vi "z.stack.configure_MD.vi"() -> ()   [LabVIEW 2012]
uses:
  GFG/GFGnumericGet.vi
  GFG/GFGbooleanGet.vi
  GFG/GFG library.lvlib
  GFG/GFGfpRefGet.vi
panel:
  in  "error in (no error)":errorcluster
  out "error out":errorcluster
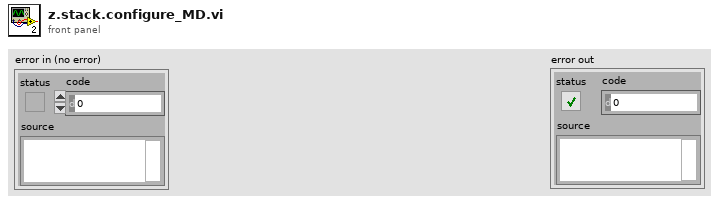
[diagram p1: front panel]
types:
  T1 = cluster{"WaveformChartRef":refnum<vi>, "DigitalRef":refnum<vi>, "ArrayRef":refnum<vi>, "TabControlRef":refnum<vi>, "EnumRef":refnum<vi>, "RingRef":refnum<vi>, "BooleanRef":refnum<vi>, "KnobRef":refnum<vi>, "SlideRef":refnum<vi>, "PathRef":refnum<vi>, "StringRef":refnum<vi>, "ComboBox":refnum<vi>, "WaveformGraphRef":refnum<vi>}
  T2 = enum8{"Enabled", "Disabled", "Disabled and Grayed Out"}
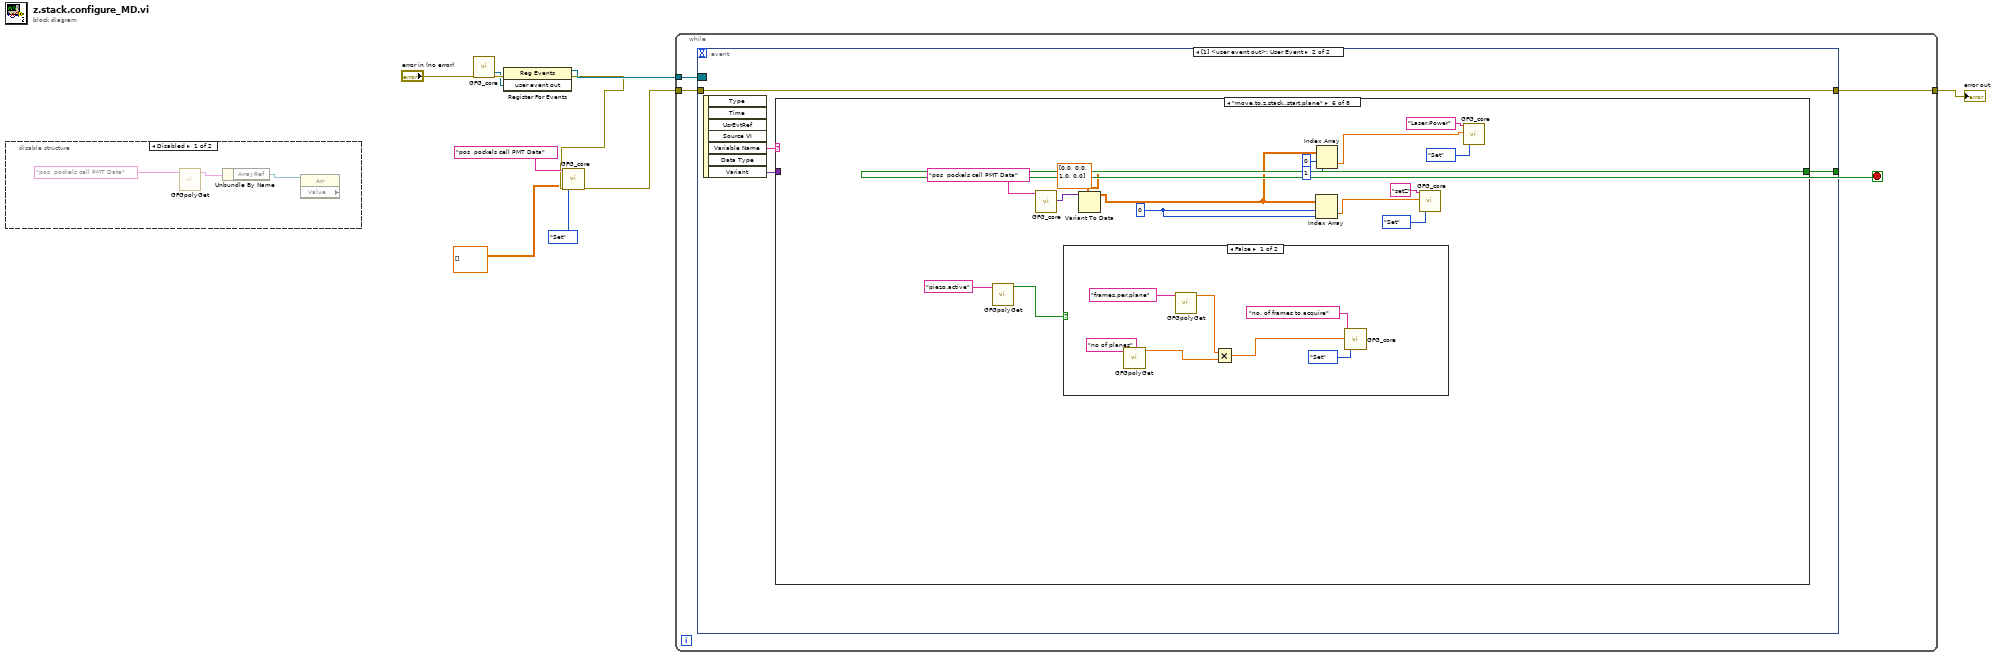
[diagram p0: block diagram]
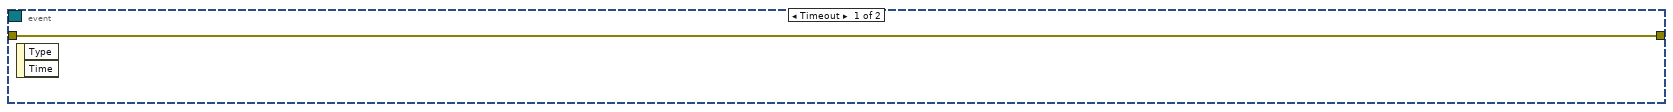
[diagram p3: hidden frame]
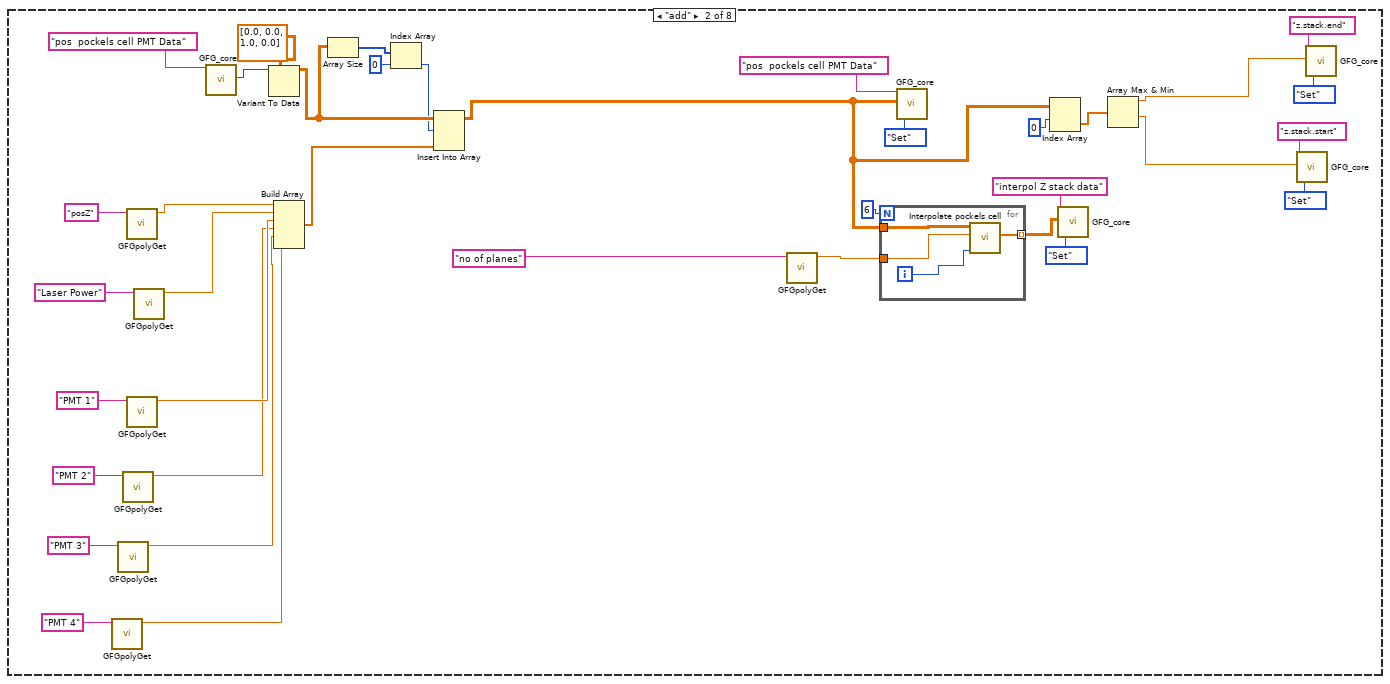
[diagram p5: hidden frame]
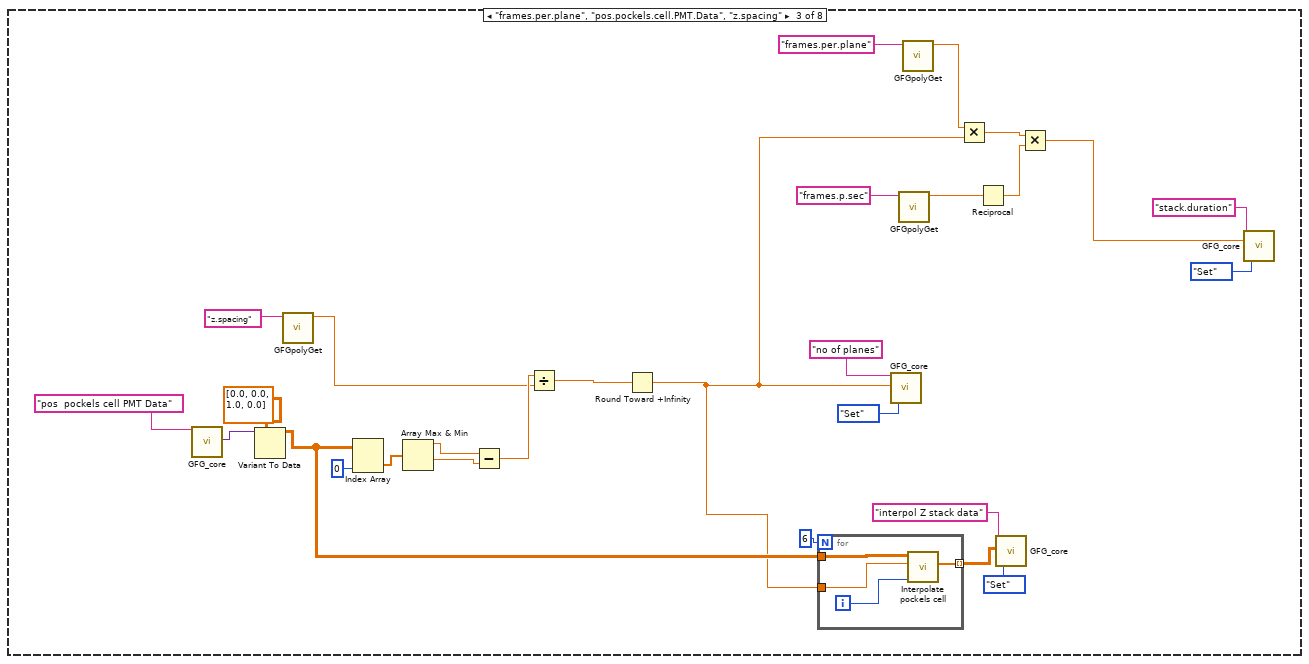
[diagram p6: hidden frame]
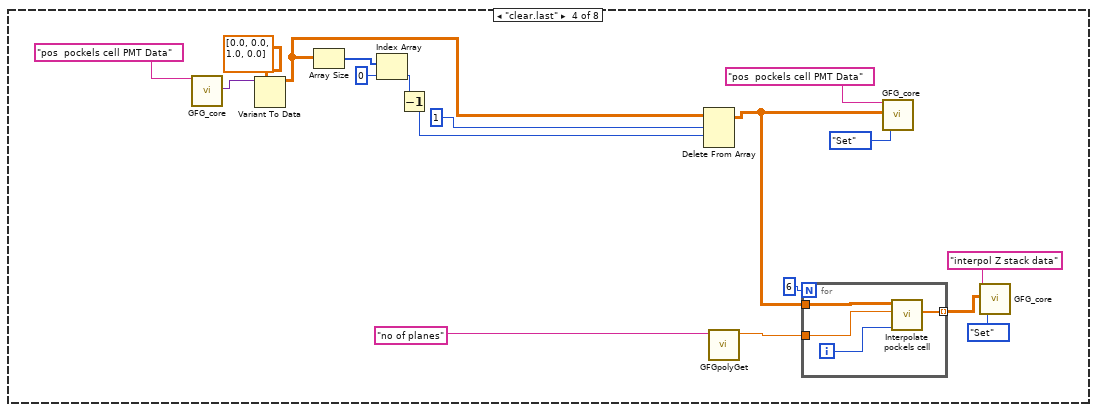
[diagram p7: hidden frame]
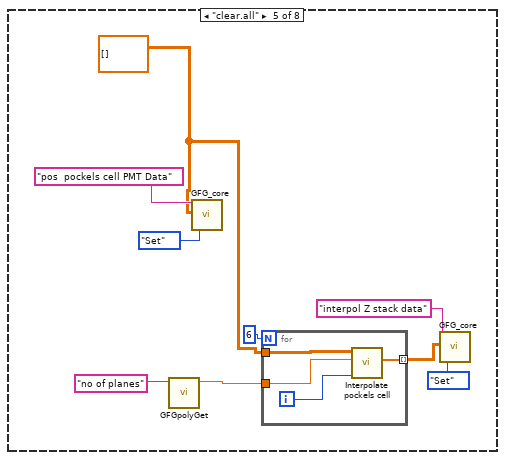
[diagram p8: hidden frame]
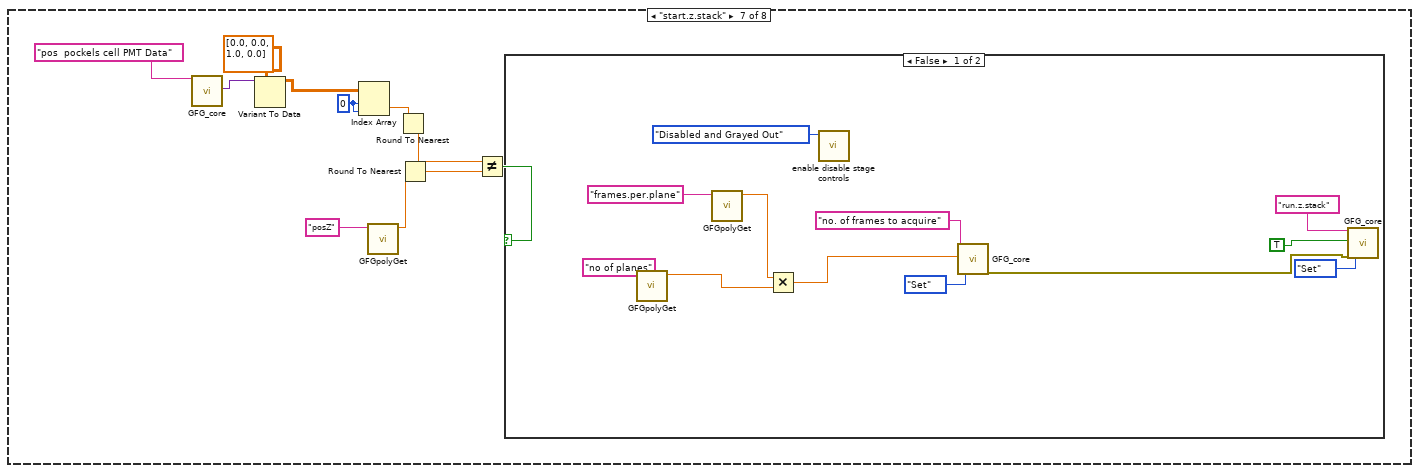
[diagram p10: hidden frame]
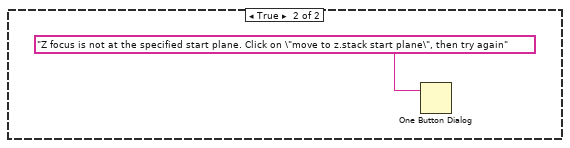
[diagram p11: hidden frame]
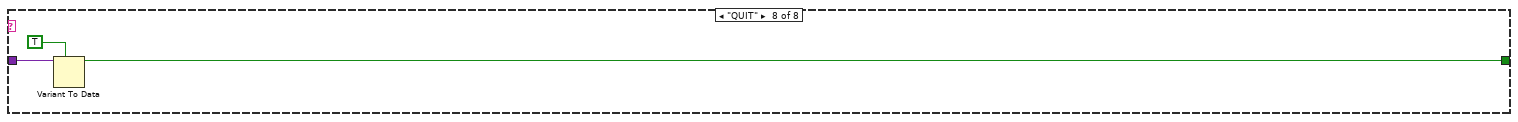
[diagram p12: hidden frame]
diagram:
  n1 = disable-structure shown="Disabled" {
    frame Disabled {
      n2 = call-poly "GFGpolyGet.vi"("Variable Name in"="pos  pockels cell PMT Data") -> ("output cluster"=w12:T1)  [unwired: 9 in, 1 out]
      n3 = Unbundle By Name(w12) -> ("ArrayRef"=w11:refnum<vi>)
      n4 = property class="Arr" props=["Value"](reference=w11) -> ()  [unwired: 1 in, 3 out]
    }
    frame Enabled {
    }
  }
  n5 = call "GFG_core.vi"("error in (no error)"="error in (no error)") -> ("user event out"=w7:refnum<user-event>, "error out"=w8:errorcluster)  [unwired: 12 in, 5 out]
  n6 = register-events(error in=w8, w7) -> (reference out=w6:refnum<event-registration>, error out=w4:errorcluster)  [unwired: 1 in]
  n7 = call "GFG_core.vi"("Variable Name in"="pos  pockels cell PMT Data", "Variant in"=dbl[][] [] ("output array"), "error in (no error)"=w4, "Action"=enum16{"Init", "Set", "Get"}."Set") -> ("error out"=w2:errorcluster)  [unwired: 9 in, 6 out]
  n8 = while {
    tunnel: w6 -> [w17]
    tunnel: w2 -> [w15]
    tunnel: [w14] -> w10
    stop <- w16 stop-if-true
    n9 = event shown="[1] <user event out>: User Event" {
      selector: w17 -> [_ _]
      dyn-events: _ -> [_ _]
      timeout: _ -> [_ _]
      tunnel: [_ w20] -> w16
      tunnel: w15 -> [w18 w19]
      tunnel: [w18 w19] -> w14
      event Timeout {
        n10 = event-data() -> ()  [unwired: 1 in, 2 out]
      }
      event User Event {
        n11 = event-data() -> ("Variable Name"=w22:string, "Variant"=w21:variant)  [unwired: 1 in, 5 out]
        n12 = case shown="\"move.to.z.stack..start.plane\"" w22 {
          tunnel: w21 -> [_ _ _ _ _ _ _ w179]
          tunnel: [_ _ _ _ _ _ _ w177] -> w20
          frame "False", Default {
          }
          frame "add" {
            n13 = call-poly "GFGpolyGet.vi"("Variable Name in"="PMT 4") -> ("Numeric"=w41:dbl)  [unwired: 9 in, 1 out]
            n14 = call-poly "GFGpolyGet.vi"("Variable Name in"="PMT 3") -> ("Numeric"=w42:dbl)  [unwired: 9 in, 1 out]
            n15 = call-poly "GFGpolyGet.vi"("Variable Name in"="PMT 2") -> ("Numeric"=w43:dbl)  [unwired: 9 in, 1 out]
            n16 = call-poly "GFGpolyGet.vi"("Variable Name in"="posZ") -> ("Numeric"=w46:dbl)  [unwired: 9 in, 1 out]
            n17 = call-poly "GFGpolyGet.vi"("Variable Name in"="PMT 1") -> ("Numeric"=w44:dbl)  [unwired: 9 in, 1 out]
            n18 = call-poly "GFGpolyGet.vi"("Variable Name in"="Laser Power") -> ("Numeric"=w45:dbl)  [unwired: 9 in, 1 out]
            n19 = call "GFG_core.vi"("Variable Name in"="pos  pockels cell PMT Data") -> ("Variant Out"=w58:variant)  [unwired: 12 in, 6 out]
            n20 = Variant To Data(type=dbl[][] [[0.0, 0.0], [1.0, 0.0]] ("pos  pockels cell PMT Data"), Variant=w58) -> (data=w56:dbl[][])  [unwired: 1 in, 1 out]
            n21 = Build Array(w46, w45, w44, w43, w42, w41) -> (w40:dbl[])
            n22 = Array Size(array=w56) -> (size(s)=w55:i32[])
            n23 = Index Array(array=w55, index=0) -> (element=w53:i32)
            n24 = Insert Into Array(array=w56, index (row)=w53, new element=w40) -> (w29:dbl[][])  [unwired: 1 in]
            n25 = call-poly "GFGpolyGet.vi"("Variable Name in"="no of planes") -> ("Numeric"=w35:dbl)  [unwired: 9 in, 1 out]
            n26 = for {
              N: 6 -> [_]
              tunnel: w29 -> [w63]
              tunnel: w35 -> [w62]
              tunnel: [w61] -> w32 mode=indexing
              i -> [w60]
              n27 = call "Interpolate pockels cell.vi"("column"=w60, "nr of planes"=w62, "Data"=w63) -> ("Interpolated Data"=w61:dbl[])  [unwired: 7 in, 1 out]
            }
            n28 = call "GFG_core.vi"("Variable Name in"="pos  pockels cell PMT Data", "Variant in"=w29, "Action"=enum16{"Init", "Set", "Get"}."Set") -> ()  [unwired: 10 in, 7 out]
            n29 = Index Array(array=w29, index (row)=0 ("disabled index (col)")) -> (element=w31:dbl[])  [unwired: 1 in]
            n30 = call "GFG_core.vi"("Variable Name in"="interpol Z stack data", "Variant in"=w32, "Action"=enum16{"Init", "Set", "Get"}."Set") -> ()  [unwired: 10 in, 7 out]
            n31 = Array Max & Min(array=w31) -> (max value=w23:dbl, min value=w24:dbl)  [unwired: 2 out]
            n32 = call "GFG_core.vi"("Variable Name in"="z.stack.start", "Variant in"=w24, "Action"=enum16{"Init", "Set", "Get"}."Set") -> ()  [unwired: 10 in, 7 out]
            n33 = call "GFG_core.vi"("Variable Name in"="z.stack.end", "Variant in"=w23, "Action"=enum16{"Init", "Set", "Get"}."Set") -> ()  [unwired: 10 in, 7 out]
          }
          frame "frames.per.plane", "pos.pockels.cell.PMT.Data", "z.spacing" {
            n34 = call "GFG_core.vi"("Variable Name in"="pos  pockels cell PMT Data") -> ("Variant Out"=w77:variant)  [unwired: 12 in, 6 out]
            n35 = Variant To Data(type=dbl[][] [[0.0, 0.0], [1.0, 0.0]] ("pos  pockels cell PMT Data"), Variant=w77) -> (data=w69:dbl[][])  [unwired: 1 in, 1 out]
            n36 = call-poly "GFGpolyGet.vi"("Variable Name in"="z.spacing") -> ("Numeric"=w67:dbl)  [unwired: 9 in, 1 out]
            n37 = Index Array(array=w69, index (col)=0 ("disabled index (col)")) -> (element=w79:dbl[])  [unwired: 1 in]
            n38 = Array Max & Min(array=w79) -> (max value=w81:dbl, min value=w82:dbl)  [unwired: 2 out]
            n39 = Subtract(x=w81, y=w82) -> (x-y=w75:dbl)
            n40 = Divide(x=w75, y=w67) -> (x/y=w74:dbl)
            n41 = Round Toward +Infinity(x=w74) -> (ceil(x): smallest int >= x=w64:dbl)
            n42 = for {
              N: 6 -> [_]
              tunnel: w69 -> [w95]
              tunnel: w64 -> [w94]
              tunnel: [w93] -> w70 mode=indexing
              i -> [w92]
              n43 = call "Interpolate pockels cell.vi"("column"=w92, "nr of planes"=w94, "Data"=w95) -> ("Interpolated Data"=w93:dbl[])  [unwired: 7 in, 1 out]
            }
            n44 = call "GFG_core.vi"("Variable Name in"="no of planes", "Variant in"=w64, "Action"=enum16{"Init", "Set", "Get"}."Set") -> ()  [unwired: 10 in, 7 out]
            n45 = call-poly "GFGpolyGet.vi"("Variable Name in"="frames.p.sec") -> ("Numeric"=w90:dbl)  [unwired: 9 in, 1 out]
            n46 = call-poly "GFGpolyGet.vi"("Variable Name in"="frames.per.plane") -> ("Numeric"=w65:dbl)  [unwired: 9 in, 1 out]
            n47 = Multiply(x=w65, y=w64) -> (x*y=w88:dbl)
            n48 = Reciprocal(x=w90) -> (1/x=w89:dbl)
            n49 = call "GFG_core.vi"("Variable Name in"="interpol Z stack data", "Variant in"=w70, "Action"=enum16{"Init", "Set", "Get"}."Set") -> ()  [unwired: 10 in, 7 out]
            n50 = Multiply(x=w88, y=w89) -> (x*y=w85:dbl)
            n51 = call "GFG_core.vi"("Variable Name in"="stack.duration", "Variant in"=w85, "Action"=enum16{"Init", "Set", "Get"}."Set") -> ()  [unwired: 10 in, 7 out]
          }
          frame "clear.last" {
            n52 = call "GFG_core.vi"("Variable Name in"="pos  pockels cell PMT Data") -> ("Variant Out"=w112:variant)  [unwired: 12 in, 6 out]
            n53 = Variant To Data(type=dbl[][] [[0.0, 0.0], [1.0, 0.0]] ("pos  pockels cell PMT Data"), Variant=w112) -> (data=w110:dbl[][])  [unwired: 1 in, 1 out]
            n54 = Array Size(array=w110) -> (size(s)=w109:i32[])
            n55 = Index Array(array=w109, index=0) -> (element=w105:i32)
            n56 = Decrement(x=w105) -> (x-1=w104:i32)
            n57 = Delete From Array(array=w110, length=1, index (row)=w104) -> (array with subset deleted=w96:dbl[][])  [unwired: 1 in, 1 out]
            n58 = call-poly "GFGpolyGet.vi"("Variable Name in"="no of planes") -> ("Numeric"=w100:dbl)  [unwired: 9 in, 1 out]
            n59 = for {
              N: 6 -> [_]
              tunnel: w96 -> [w117]
              tunnel: w100 -> [w116]
              tunnel: [w115] -> w97 mode=indexing
              i -> [w114]
              n60 = call "Interpolate pockels cell.vi"("column"=w114, "nr of planes"=w116, "Data"=w117) -> ("Interpolated Data"=w115:dbl[])  [unwired: 7 in, 1 out]
            }
            n61 = call "GFG_core.vi"("Variable Name in"="pos  pockels cell PMT Data", "Variant in"=w96, "Action"=enum16{"Init", "Set", "Get"}."Set") -> ()  [unwired: 10 in, 7 out]
            n62 = call "GFG_core.vi"("Variable Name in"="interpol Z stack data", "Variant in"=w97, "Action"=enum16{"Init", "Set", "Get"}."Set") -> ()  [unwired: 10 in, 7 out]
          }
          frame "clear.all" {
            w118 = dbl[][] [] ("output array")
            n63 = call-poly "GFGpolyGet.vi"("Variable Name in"="no of planes") -> ("Numeric"=w122:dbl)  [unwired: 9 in, 1 out]
            n64 = call "GFG_core.vi"("Variable Name in"="pos  pockels cell PMT Data", "Variant in"=w118, "Action"=enum16{"Init", "Set", "Get"}."Set") -> ()  [unwired: 10 in, 7 out]
            n65 = for {
              N: 6 -> [_]
              tunnel: w118 -> [w130]
              tunnel: w122 -> [w129]
              tunnel: [w128] -> w119 mode=indexing
              i -> [w127]
              n66 = call "Interpolate pockels cell.vi"("column"=w127, "nr of planes"=w129, "Data"=w130) -> ("Interpolated Data"=w128:dbl[])  [unwired: 7 in, 1 out]
            }
            n67 = call "GFG_core.vi"("Variable Name in"="interpol Z stack data", "Variant in"=w119, "Action"=enum16{"Init", "Set", "Get"}."Set") -> ()  [unwired: 10 in, 7 out]
          }
          frame "move.to.z.stack..start.plane" {
            w142 = 0 ("index (row)")
            n68 = call-poly "GFGpolyGet.vi"("Variable Name in"="piezo.active") -> ("Boolean"=w137:bool)  [unwired: 10 in]
            n69 = call "GFG_core.vi"("Variable Name in"="pos  pockels cell PMT Data") -> ("Variant Out"=w144:variant)  [unwired: 12 in, 6 out]
            n70 = case shown="False" w137 {
              frame False {
                n71 = call-poly "GFGpolyGet.vi"("Variable Name in"="no of planes") -> ("Numeric"=w151:dbl)  [unwired: 9 in, 1 out]
                n72 = call-poly "GFGpolyGet.vi"("Variable Name in"="frames.per.plane") -> ("Numeric"=w149:dbl)  [unwired: 9 in, 1 out]
                n73 = Multiply(x=w149, y=w151) -> (x*y=w152:dbl)
                n74 = call "GFG_core.vi"("Variable Name in"="no. of frames to acquire", "Variant in"=w152, "Action"=enum16{"Init", "Set", "Get"}."Set") -> ()  [unwired: 10 in, 7 out]
              }
              frame True {
              }
            }
            n75 = Variant To Data(type=dbl[][] [[0.0, 0.0], [1.0, 0.0]] ("pos  pockels cell PMT Data"), Variant=w144) -> (data=w134:dbl[][])  [unwired: 1 in, 1 out]
            n76 = Index Array(array=w134, index (row)=w142, index (col)=w142) -> (element=w139:dbl)
            n77 = Index Array(array=w134, index (row)=0, index (col)=1 ("disabled index (col)")) -> (element=w131:dbl)
            n78 = call "GFG_core.vi"("Variable Name in"="setZ", "Variant in"=w139, "Action"=enum16{"Init", "Set", "Get"}."Set") -> ()  [unwired: 10 in, 7 out]
            n79 = call "GFG_core.vi"("Variable Name in"="Laser.Power", "Variant in"=w131, "Action"=enum16{"Init", "Set", "Get"}."Set") -> ()  [unwired: 10 in, 7 out]
          }
          frame "start.z.stack" {
            w159 = 0 ("index (row)")
            n80 = call "GFG_core.vi"("Variable Name in"="pos  pockels cell PMT Data") -> ("Variant Out"=w162:variant)  [unwired: 12 in, 6 out]
            n81 = Variant To Data(type=dbl[][] [[0.0, 0.0], [1.0, 0.0]] ("pos  pockels cell PMT Data"), Variant=w162) -> (data=w160:dbl[][])  [unwired: 1 in, 1 out]
            n82 = Index Array(array=w160, index (row)=w159, index (col)=w159) -> (element=w157:dbl)
            n83 = call-poly "GFGpolyGet.vi"("Variable Name in"="posZ") -> ("Numeric"=w156:dbl)  [unwired: 9 in, 1 out]
            n84 = Round To Nearest(number=w157) -> (nearest integer value=w154:dbl)
            n85 = Round To Nearest(number=w156) -> (nearest integer value=w153:dbl)
            n86 = Not Equal?(x=w154, y=w153) -> (x != y?=w155:bool)
            n87 = case shown="False" w155 {
              frame False {
                n88 = call-poly "GFGpolyGet.vi"("Variable Name in"="no of planes") -> ("Numeric"=w170:dbl)  [unwired: 9 in, 1 out]
                n89 = call-poly "GFGpolyGet.vi"("Variable Name in"="frames.per.plane") -> ("Numeric"=w168:dbl)  [unwired: 9 in, 1 out]
                n90 = Multiply(x=w168, y=w170) -> (x*y=w171:dbl)
                n91 = call "enable disable stage controls.vi"("Disabled"=T2."Disabled and Grayed Out") -> ()  [unwired: 11 in]
                n92 = call "GFG_core.vi"("Variable Name in"="no. of frames to acquire", "Variant in"=w171, "Action"=enum16{"Init", "Set", "Get"}."Set") -> ("error out"=w164:errorcluster)  [unwired: 10 in, 6 out]
                n93 = call "GFG_core.vi"("Variable Name in"="run.z.stack", "Variant in"=TRUE, "error in (no error)"=w164, "Action"=enum16{"Init", "Set", "Get"}."Set") -> ()  [unwired: 9 in, 7 out]
              }
              frame True {
                n94 = One Button Dialog(message="Z focus is not at the specified start plane. Click on \"move to z.stack start plane\", then try again") -> ()  [unwired: 1 in, 1 out]
              }
            }
          }
          frame "QUIT" {
            n95 = Variant To Data(type=TRUE ("want seconds? (F)"), Variant=w179) -> (data=w177:bool)  [unwired: 1 in, 1 out]
          }
        }
      }
    }
  }
  "error out" <- w10
